vi "scan_get_duration.vi"(5 "total_steps":u32, 7 "current_iteration":u32, 8 "error in (no error)":errorcluster, 10 "current_position":dbl, 11 "scan_panel in":refnum<class "scan_panel.lvclass">) -> (0 "error out":errorcluster, 2 "time_remaining":string, 3 "scan_panel out":refnum<class "scan_panel.lvclass">)   [LabVIEW 2015, in "scan_panel.lvclass"]
uses:
  scan_panel.lvclass
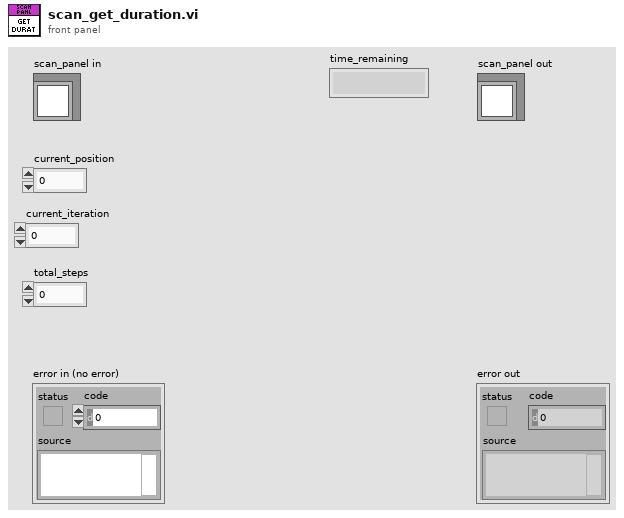
[diagram p1: front panel]
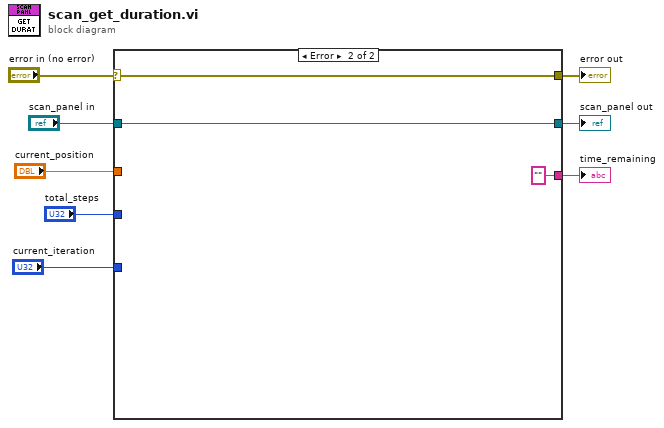
[diagram p0: block diagram]
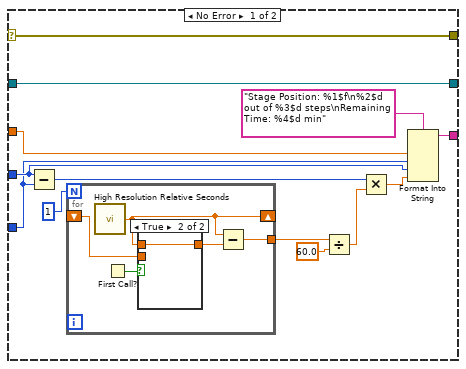
[diagram p2: hidden frame]
diagram:
  n1 = case shown="Error" "error in (no error)" {
    selector: "error in (no error)" -> [w20 w31]
    tunnel: [w20 w31] -> w7
    tunnel: [w21 w30] -> w5
    tunnel: "scan_panel in" -> [w21 w30]
    tunnel: "current_position" -> [w18 _]
    tunnel: "current_iteration" -> [w13 _]
    tunnel: "total_steps" -> [w14 _]
    tunnel: [w9 ""] -> w1
    frame No Error {
      n2 = Subtract(x=w14, y=w13) -> (x-y=w12:u32)
      n3 = for {
        N: 1 -> [_]
        shift-right: [w23] -> _
        shift-left: _ -> [w25]
        tunnel: [w26] -> w16
        n4 = call <vilib>:"High Resolution Relative Seconds.vi"() -> ("relative seconds"=w23:dbl)
        n5 = First Call?() -> (First Call?: T/F=w22:bool)
        n6 = case shown="True" w22 {
          tunnel: w25 -> [w27 _]
          tunnel: [w27 w28] -> w24
          tunnel: w23 -> [_ w28]
          frame False {
          }
          frame True {
          }
        }
        n7 = Subtract(x=w23, y=w24) -> (x-y=w26:dbl)
      }
      n8 = Divide(x=w16, y=60.0) -> (x/y=w11:dbl)
      n9 = Multiply(x=w12, y=w11) -> (x*y=w10:dbl)
      n10 = Format Into String(format string="Stage Position: %1$f\n%2$d out of %3$d steps\nRemaining Time: %4$d min", w18, w13, w14, w10) -> (resulting string=w9:string)  [unwired: 2 in, 1 out]
    }
    frame Error {
    }
  }
  "error out" <- w7
  "scan_panel out" <- w5
  "time_remaining" <- w1
